vi "Generate Ramp.vi"(8 "error in (no error)":errorcluster, 10 "Settings":T1) -> (0 "error out":errorcluster)   [LabVIEW 2020, in "High Level PSU With Tests.lvlib"]
uses:
  High Level PSU With Tests.lvlib
  Ramp Voltage/Ramp Settings.ctl
  Ramp Voltage/Ramp Voltage.lvclass
  PSU/PSU.lvclass
  C:/Git/astemes-gdevcon-2022/PSU Demo/High Level PSU With Tests/Voltage Output/Voltage Output.lvclass
  Ramp Voltage/Ramp Voltage.lvclass/Ramp Voltage.ctl
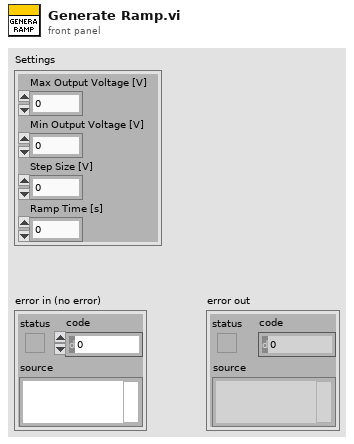
[diagram p1: front panel]
types:
  T1 = typedef "High Level PSU With Tests.lvlib/Ramp Voltage.lvclass/Ramp Settings.ctl" = cluster{"Max Output Voltage [V]":dbl, "Min Output Voltage [V]":dbl, "Step Size [V]":dbl, "Ramp Time [s]":dbl}
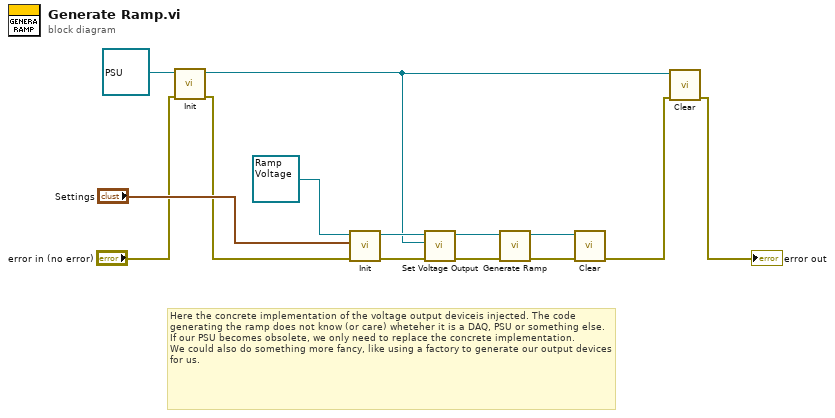
[diagram p0: block diagram]
diagram:
  # "Here the concrete implementation of the voltage output deviceis injected. The code generating the ramp does not know (or care) wheteher it is a DAQ, PSU or something else. If our PSU becomes obsolete, we only need to replace the concrete implementation. \nWe could also do something more fancy, like using a factory to generate our output devices for us."
  n1 = call "Init.vi"("error in (no error)"="error in (no error)", "PSU in"=refnum<class "PSU.lvclass"> refnum) -> ("error out"=w2:errorcluster, "PSU out"=w6:refnum<class "PSU.lvclass">)  [unwired: 8 in]
  n2 = call "Init.vi"("error in (no error)"=w2, "Settings"="Settings", "Ramp Voltage In"=refnum<class "Ramp Voltage.lvclass"> refnum) -> ("error out"=w1:errorcluster, "Ramp Voltage Out"=w14:refnum<class "Ramp Voltage.lvclass">)  [unwired: 7 in]
  n3 = call "Set Voltage Output.vi"("error in (no error)"=w1, "Voltage Output"=w6, "Ramp Voltage In"=w14) -> ("error out"=w12:errorcluster, "Ramp Voltage Out"=w13:refnum<class "Ramp Voltage.lvclass">)  [unwired: 7 in]
  n4 = call "Generate Ramp.vi"("error in (no error)"=w12, "Ramp Use Case In"=w13) -> ("error out"=w10:errorcluster, "Ramp Use Case Out"=w11:refnum<class "Ramp Voltage.lvclass">)  [unwired: 8 in]
  n5 = call "Clear.vi"("error in (no error)"=w10, "Ramp Use Case in"=w11) -> ("error out"=w5:errorcluster)  [unwired: 8 in, 1 out]
  n6 = call "Clear.vi"("error in (no error)"=w5, "PSU in"=w6) -> ("error out"=→"error out":errorcluster)  [unwired: 8 in, 1 out]
